vi "test_ParseSolutionFile_TestAssetSolutions.vi"() -> (3 "Pass?":bool)   [LabVIEW 2019, in "Tests.SolutionBuilder.lvlib"]
uses:
  Tests.SolutionBuilder.lvlib
  SolutionBuilder/SolutionBuilder.lvclass
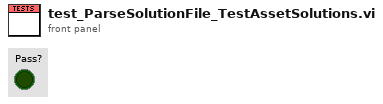
[diagram p1: front panel]
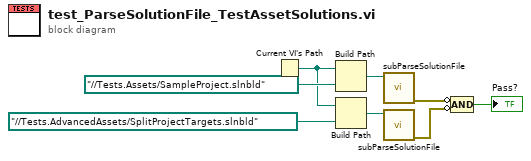
[diagram p0: block diagram]
diagram:
  n1 = Current VI's Path() -> (path=w1:path)
  n2 = Build Path(base path=w1, name or relative path=path "../../Tests.Assets/SampleProject.slnbld" ("Path")) -> (appended path=w6:path)
  n3 = Build Path(base path=w1, name or relative path=path "../../Tests.AdvancedAssets/SplitProjectTargets.slnbld" ("Path")) -> (appended path=w4:path)
  n4 = call "subParseSolutionFile.vi"("Solution file"=w6) -> ("error out"=w5:errorcluster)  [unwired: 7 in, 3 out]
  n5 = call "subParseSolutionFile.vi"("Solution file"=w4) -> ("error out"=w2:errorcluster)  [unwired: 7 in, 3 out]
  n6 = Compound Arithmetic op=AND(invert w5, invert w2) -> (→"Pass?":bool)
